vi "DBL[1D]小数与整数（商与余数）.vi"(11 "输入":dbl[](array[numeric])) -> (2 "小数部分":dbl[](array[numeric]), 3 "整数部分":dbl[](array[numeric]))   [LabVIEW 2012]
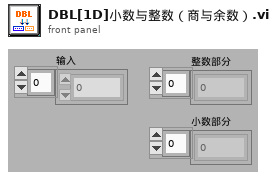
[diagram p1: front panel]
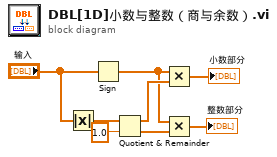
[diagram p0: block diagram]
diagram:
  n1 = Absolute Value(x="输入") -> (abs(x)=w5:dbl[])
  n2 = Sign(1:"输入") -> (0:w1:dbl[])
  n3 = Quotient & Remainder(x=w5, y=1.0) -> (x-y*floor(x/y)=w7:dbl[], floor(x/y)=w6:dbl[])
  n4 = Multiply(x=w1, y=w7) -> (x*y=→"小数部分":dbl[])
  n5 = Multiply(x=w1, y=w6) -> (x*y=→"整数部分":dbl[])
